vi "Gasflasche Text in Cluster.vi"(10 "Gasflasche Text Array":T1[](array[typedef])) -> (2 "Gasflasche":T2={"Gasflasche"={"Gasname für die Auswahl"="", "Chargennummer"="", "Ablaufdatum"=timestamp(0 s since 1904-01-01)}, "Trägergas"="N2", "Komponenten"=[]} {"Gasflasche"."Ablaufdatum" format="%<%d.%m.%Y>T"; "Komponenten"."Konzentration IST" format="%#.4f"; "Komponenten"."Genauigkeit" format="%#.1f"})   [LabVIEW 2020, in "System Einstellungen V2.lvlib"]
uses:
  System Einstellungen V2.lvlib
  Gasflasche gesamt.ctl
  Gasflasche.ctl
  Traegergas.ctl
  Gasflaschenkomponente.ctl
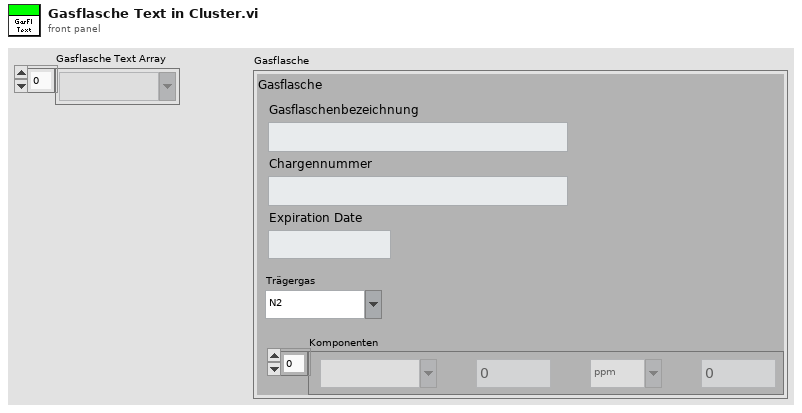
[diagram p1: front panel]
types:
  T1 = typedef "System Einstellungen V2.lvlib/Traegergas.ctl" = string
  T2 = typedef "System Einstellungen V2.lvlib/Gasflasche gesamt.ctl" = cluster{"Gasflasche":T3, "Trägergas":T1, "Komponenten":T4[]}
  T3 = typedef "System Einstellungen V2.lvlib/Gasflasche.ctl" = cluster{"Gasname für die Auswahl":string, "Chargennummer":string, "Ablaufdatum":timestamp}
  T4 = typedef "System Einstellungen V2.lvlib/Gasflaschenkomponente.ctl" = cluster{"Gasauswahl":string, "Konzentration IST":dbl, "Einheit":string, "Genauigkeit":dbl}
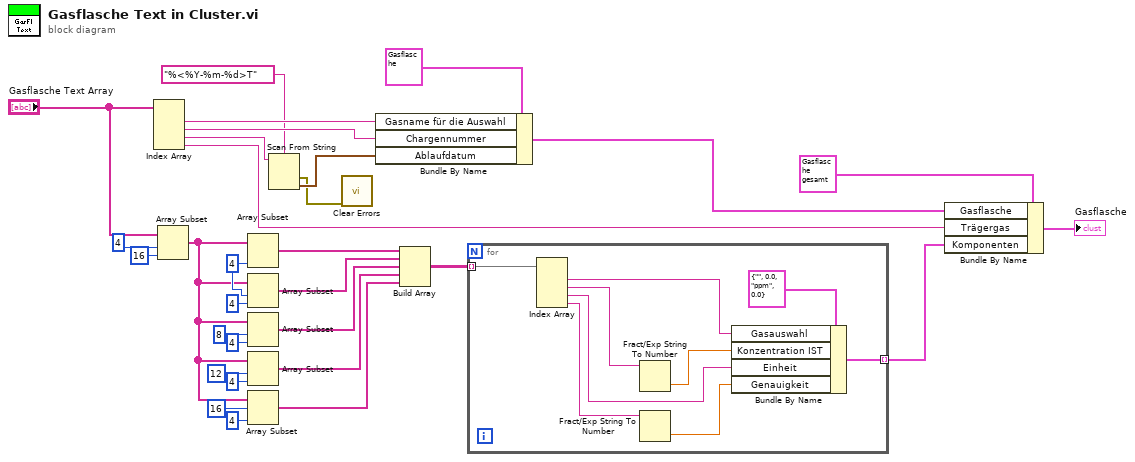
[diagram p0: block diagram]
diagram:
  w20 = 4 ("Länge")
  n1 = Index Array(array="Gasflasche Text Array") -> (element #1=w26:T1, element #2=w25:T1, element #3=w3:T1, element #4=w4:T1)  [unwired: 4 in]
  n2 = Array Subset(array="Gasflasche Text Array", index=4 ("Länge"), length=16 ("Länge")) -> (w15:T1[])
  n3 = Array Subset(array=w15, length=w20) -> (w11:T1[])  [unwired: 1 in]
  n4 = Array Subset(array=w15, index=w20, length=4 ("Länge")) -> (w10:T1[])
  n5 = Array Subset(array=w15, index=8 ("Index"), length=4 ("Länge")) -> (w9:T1[])
  n6 = Array Subset(array=w15, index=12 ("Index"), length=4 ("Länge")) -> (w8:T1[])
  n7 = Array Subset(array=w15, index=16 ("Index"), length=4 ("Länge")) -> (w7:T1[])
  n8 = Scan From String(format string="%<%Y-%m-%d>T" ("Format-String"), input string=w3) -> (error out=w1:errorcluster, output 1=w24:timestamp)  [unwired: 3 in, 2 out]
  n9 = call <vilib>:"Clear Errors.vi"("error in (no error)"=w1) -> ()  [unwired: 5 in, 2 out]
  n10 = Bundle By Name(cluster=T3 {"Gasname für die Auswahl"="CH4", "Chargennummer"="D15442589", "Ablaufdatum"=timestamp(0 s since 1904-01-01)} ("Gasflasche"), "Gasname für die Auswahl"=w26, "Chargennummer"=w25, "Ablaufdatum"=w24) -> (w28:T3)
  n11 = Build Array(w11, w10, w9, w8, w7) -> (w6:T1[][])
  n12 = for {
    tunnel: w6 -> [w37] mode=indexing
    tunnel: [w38] -> w5 mode=indexing
    n13 = Index Array(array=w37) -> (element #1=w36:T1, element #2=w33:T1, element #3=w32:T1, element #4=w31:T1)  [unwired: 4 in]
    n14 = Fract/Exp String To Number(string=w33) -> (number=w35:dbl)  [unwired: 3 in, 1 out]
    n15 = Fract/Exp String To Number(string=w31) -> (number=w34:dbl)  [unwired: 3 in, 1 out]
    n16 = Bundle By Name(cluster=T4 {"Gasauswahl"="", "Konzentration IST"=0.0, "Einheit"="ppm", "Genauigkeit"=0.0} ("Komponenten"), "Gasauswahl"=w36, "Konzentration IST"=w35, "Einheit"=w32, "Genauigkeit"=w34) -> (w38:T4)
  }
  n17 = Bundle By Name(cluster=T2 {"Gasflasche"={"Gasname für die Auswahl"="", "Chargennummer"="", "Ablaufdatum"=timestamp(0 s since 1904-01-01)}, "Trägergas"="N2", "Komponenten"=[]} ("Gasflasche"), "Gasflasche"=w28, "Trägergas"=w4, "Komponenten"=w5) -> (→"Gasflasche":T2)
